vi "getMIData.vi"(11 "MIILC in":refnum<class "MIILC.lvclass">) -> (2 "MIData":T1 {"Responses"."Inclination" items=["OK", "IllegalFunction", "IllegalDataAddress", "IllegalDataValue", "SlaveDeviceFailure", "Acknowledge", "SlaveDeviceBusy", "NegativeAcknowledge", "MemoryParityError", "GatewayPathUnavailable", "GatewayTargetDeviceFailedToRespond"]}, 3 "MIILC out":refnum<class "MIILC.lvclass">)   [LabVIEW 2016, in "RTMIILC.lvlib" / "MIILC.lvclass"]
uses:
  MIILC.lvclass
  DataTypes/MIData.ctl
  DataTypes/MIConstants.ctl
  DataTypes/MITelemetry.ctl
  DataTypes/MIResponses.ctl
  Common_RT_Modbus/DataTypes/ExceptionCodes.ctl
  DataTypes/MITimings.ctl
  MIILC.lvclass/MIILC.ctl
  RTMIILC.lvlib
  Common_RT_Modbus/RTModbus.lvlib
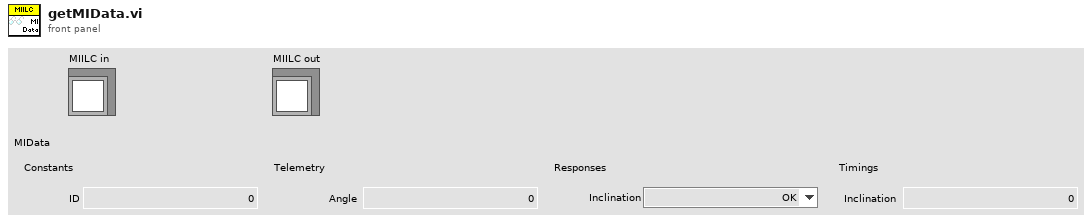
[diagram p1: front panel]
types:
  T1 = typedef "RTMIILC.lvlib/MIData.ctl" = cluster{"Constants":T2, "Telemetry":T3, "Responses":T4, "Timings":T6}
  T2 = typedef "RTMIILC.lvlib/MIConstants.ctl" = cluster{"ID":i16}
  T3 = typedef "RTMIILC.lvlib/MITelemetry.ctl" = cluster{"Angle":sgl}
  T4 = typedef "RTMIILC.lvlib/MIResponses.ctl" = cluster{"Inclination":T5}
  T5 = typedef "RTModbus.lvlib/ExceptionCodes.ctl" = u16
  T6 = typedef "RTMIILC.lvlib/MITimings.ctl" = cluster{"Inclination":u32}
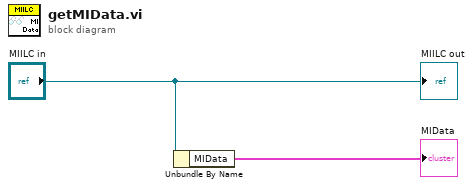
[diagram p0: block diagram]
diagram:
  n1 = Unbundle By Name("MIILC in") -> ("MIData"=→"MIData":T1)
  "MIILC out" <- "MIILC in"
